vi "_replace stopArr element.vi"(9 "new element/subarray":bool, 10 "index":i16, 11 "Array in":bool[](array[boolean])) -> (3 "Array out":bool[](array[boolean]))   [LabVIEW 2017, in "GSTOP.lvlib"]
uses:
  GSTOP.lvlib
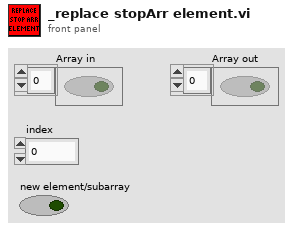
[diagram p1: front panel]
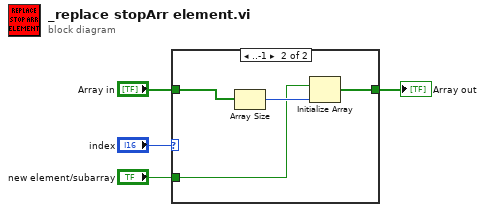
[diagram p0: block diagram]
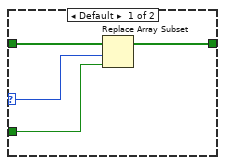
[diagram p2: hidden frame]
diagram:
  n1 = case shown="..-1" "index" {
    selector: "index" -> [w7 _]
    tunnel: "Array in" -> [w8 w12]
    tunnel: [w6 w10] -> w3
    tunnel: "new element/subarray" -> [w5 w9]
    frame Default {
      n2 = Replace Array Subset(array=w8, new element=w5, index=w7) -> (w6:bool[])
    }
    frame ..-1 {
      n3 = Array Size(array=w12) -> (size(s)=w11:i32)
      n4 = Initialize Array(w9, w11) -> (w10:bool[])
    }
  }
  "Array out" <- w3
